vi "BoP Model Control.vi"() -> ()   [LabVIEW 2017]
uses:
  <vilib>/Platform/TimedLoop/XDataNode/timing_clust.ctl
  <vilib>/Platform/TimedLoop/XDataNode/nitl_modes.ctl
  <vilib>/Platform/TimedLoop/XDataNode/wakeup.ctl
  <vilib>/Model Interface Toolkit/Model Interface Toolkit.lvclass/Model Interface Toolkit.ctl
  <vilib>/Model Interface Toolkit/Model Update.vi
  <vilib>/Model Interface Toolkit/Tick Model.vi
  <vilib>/Model Interface Toolkit/Probe Signals.vi
  <vilib>/Model Interface Toolkit/Multirate/Dispatch Model Tasks.vi
  <vilib>/Model Interface Toolkit/Call Model Start Routine.vi
  <vilib>/Model Interface Toolkit/Handle Error.vi
  <vilib>/Model Interface Toolkit/Multirate/Wait on Tasks.vi
  <vilib>/Model Interface Toolkit/Check Error.vi
  <vilib>/Model Interface Toolkit/Generate Error Cluster.vi
  <vilib>/Platform/TimedLoop/scheduler/LVUserAPI/Fire Software-Triggered Timing Source.vi
  <vilib>/Platform/TimedLoop/XDataNode/XDataNode.xnode
  <vilib>/Model Interface Toolkit/Model Interface Toolkit.lvclass
  <vilib>/Platform/TimedLoop/XDataNode/XDNodeRunTimeDep.lvlib
panel:
  in  "Stop":bool=TRUE
  in  "Model Path":path
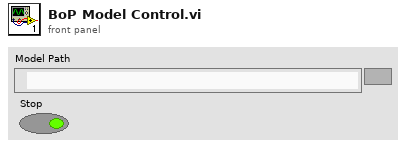
[diagram p1: front panel]
types:
  T1 = typedef "XDNodeRunTimeDep.lvlib/timing_clust.ctl" = cluster{"Expected End [f-1]":u64, "Actual End [f-1]":u64, "Finished Late? [f-1]":bool, "Expected End [i-1]":u64, "Actual End [i-1]":u64, "Finished Late? [i-1]":bool, "Expected Start [i]":u64, "Actual Start [i]":u64, "Expected Start [f]":u64, "Actual Start [f]":u64, "Source Name":string, "Structure Name":string, "Period":i64, "Deadline":i64, "Offset":i64, "Start":i64, "Priority":i32, "Timeout":i32, "Mode":T2, "Wakeup Reason":T3, "Error":errorcluster, "Source Type":string, "Secondary Source Type":string, "Global End Time":u64, "Global Start Time":u64, "Frame Duration":u64, "Iteration Duration":u64, "Assigned CPU":i32, "I/O Scan Engine Mode":u32}
  T2 = typedef "XDNodeRunTimeDep.lvlib/nitl_modes.ctl" = enum32{"No Change", "Process missed periods, maintain original phase", "Discard missed periods, maintain original phase", "Process missed periods, ignore original phase", "Discard missed periods, ignore original phase"}
  T3 = typedef "XDNodeRunTimeDep.lvlib/wakeup.ctl" = enum32{"Normal", "Aborted", "Asynchronous wakeup", "Timing source error", "Timed loop error", "Timeout"}
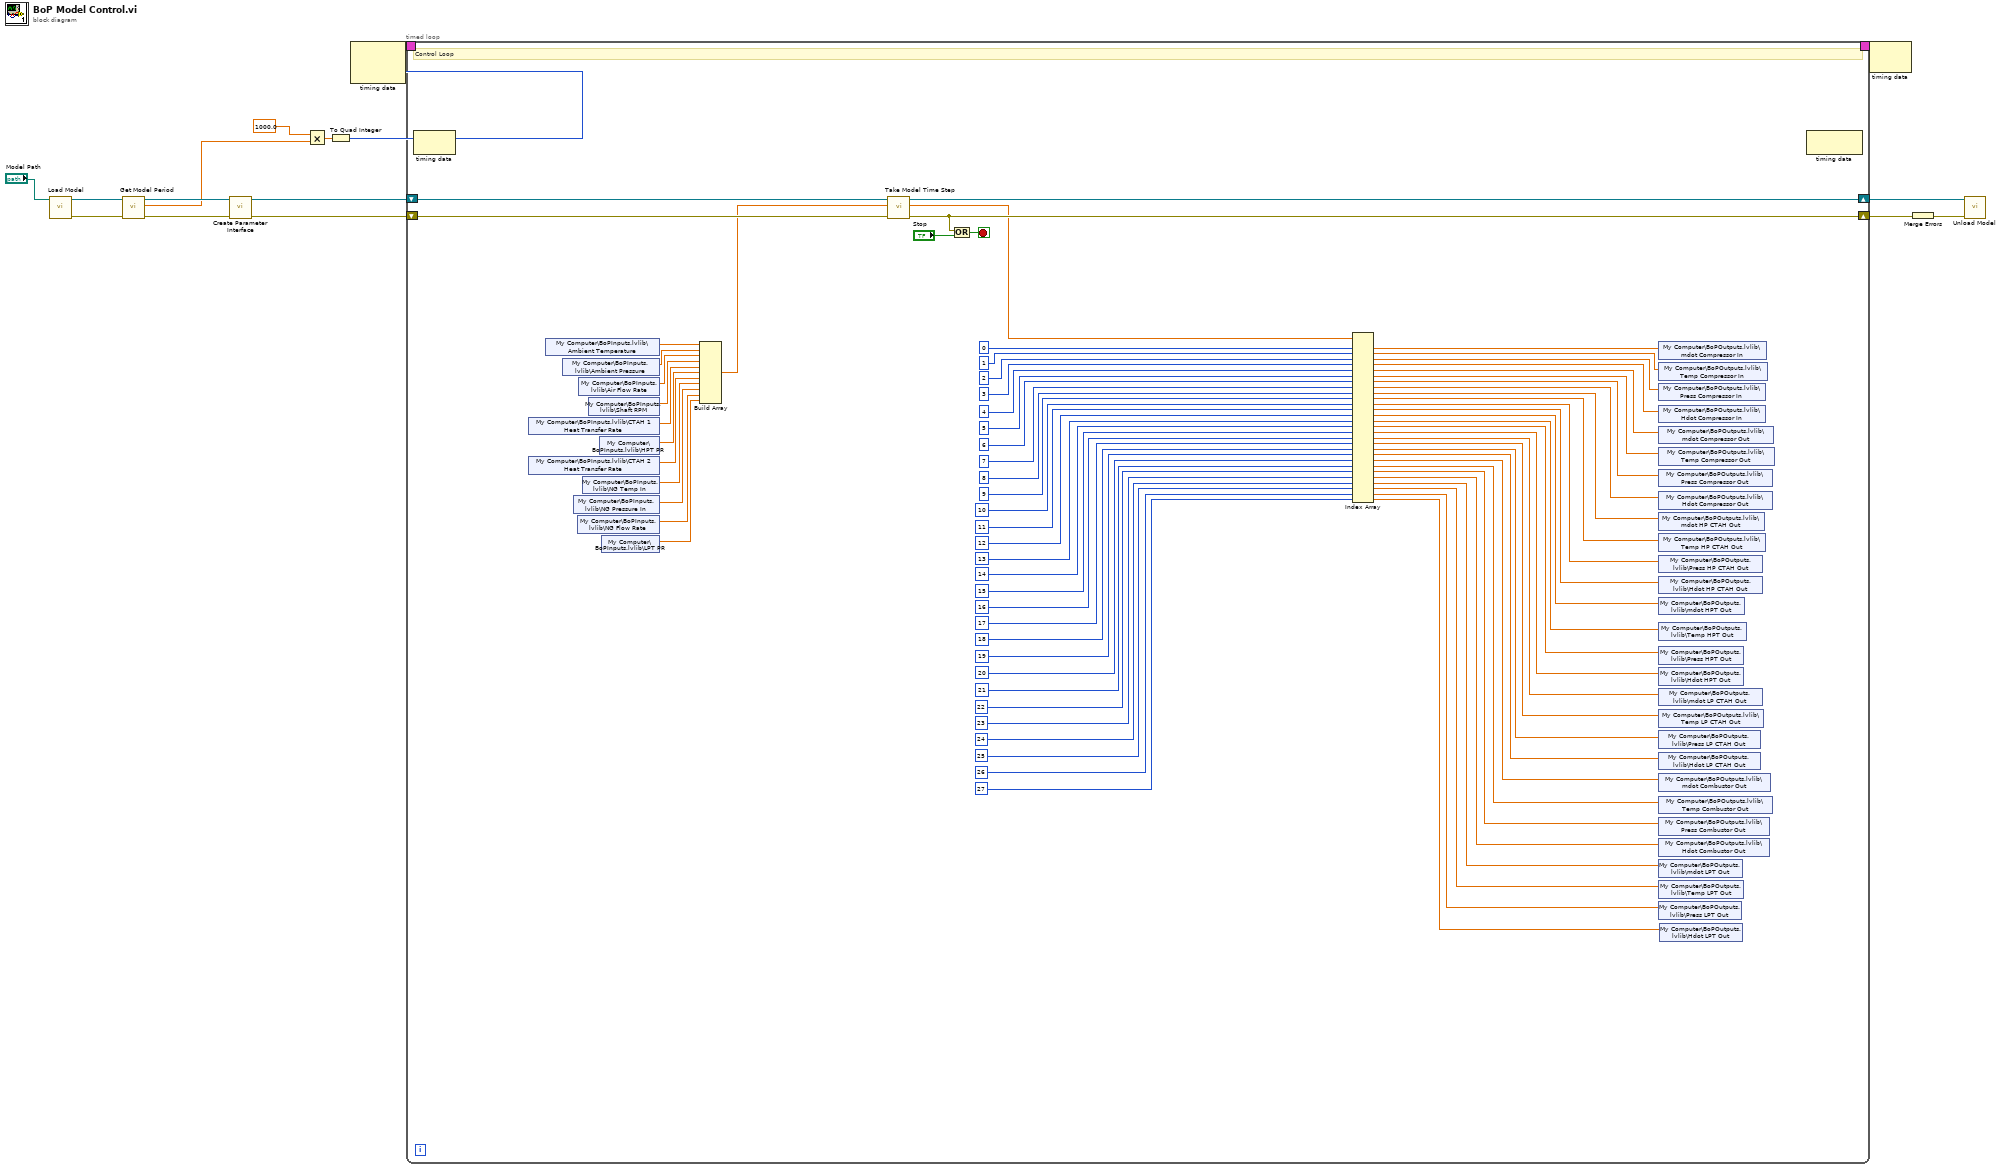
[diagram p0: block diagram]
diagram:
  n1 = call <vilib>:"Load Model.vi"("Model Path"="Model Path") -> ("error out"=w10:errorcluster, "Model out"=w13:refnum<class "Model Interface Toolkit.lvclass">)  [unwired: 9 in]
  n2 = call <vilib>:"Get Model Period.vi"("error in"=w10, "Model in"=w13) -> ("error out"=w9:errorcluster, "Model Period (s)"=w3:dbl, "Model out"=w12:refnum<class "Model Interface Toolkit.lvclass">)  [unwired: 7 in]
  n3 = call <vilib>:"Create Parameter Interface.vi"("error in"=w9, "Model in"=w12) -> ("error out"=w8:errorcluster, "Model out"=w11:refnum<class "Model Interface Toolkit.lvclass">)  [unwired: 7 in, 1 out]
  n4 = Multiply(x=1000.0, y=w3) -> (x*y=w2:dbl)
  n5 = To Quad Integer(1:w2) -> (0:w1:i64)
  n6 = node-c288(w1) -> (w15:T1)  [unwired: 1 in]
  n7 = timed-loop {
    timing: w15 -> [_]
    timing-out: [_] -> w14
    shift-right: [w90] -> w7
    shift-left: w11 -> [w91]
    shift-right: [w87] -> w6
    shift-left: w8 -> [w89]
    stop <- w88 stop-if-true
    # "Control Loop"
    n8 = node-c288() -> ()  [unwired: 1 in, 1 out]
    n9 = shared-variable "My Computer\\BoPInputs.lvlib\\CTAH 1 Heat Transfer Rate"() -> (w79:sgl)  [unwired: 1 in, 1 out]
    n10 = shared-variable "My Computer\\BoPInputs.lvlib\\CTAH 2 Heat Transfer Rate"() -> (w77:sgl)  [unwired: 1 in, 1 out]
    n11 = shared-variable "My Computer\\BoPInputs.lvlib\\Ambient Temperature"() -> (w83:sgl)  [unwired: 1 in, 1 out]
    n12 = shared-variable "My Computer\\BoPInputs.lvlib\\Ambient Pressure"() -> (w82:sgl)  [unwired: 1 in, 1 out]
    n13 = shared-variable "My Computer\\BoPInputs.lvlib\\NG Pressure In"() -> (w75:sgl)  [unwired: 1 in, 1 out]
    n14 = shared-variable "My Computer\\BoPInputs.lvlib\\NG Flow Rate"() -> (w74:sgl)  [unwired: 1 in, 1 out]
    n15 = shared-variable "My Computer\\BoPInputs.lvlib\\Air Flow Rate"() -> (w81:sgl)  [unwired: 1 in, 1 out]
    n16 = shared-variable "My Computer\\BoPInputs.lvlib\\NG Temp In"() -> (w76:sgl)  [unwired: 1 in, 1 out]
    n17 = shared-variable "My Computer\\BoPInputs.lvlib\\Shaft RPM"() -> (w80:sgl)  [unwired: 1 in, 1 out]
    n18 = shared-variable "My Computer\\BoPInputs.lvlib\\HPT PR"() -> (w78:sgl)  [unwired: 1 in, 1 out]
    n19 = shared-variable "My Computer\\BoPInputs.lvlib\\LPT PR"() -> (w73:sgl)  [unwired: 1 in, 1 out]
    n20 = Build Array(w83, w82, w81, w80, w79, w78, w77, w76, w75, w74, w73) -> (w86:sgl[])
    n21 = call <vilib>:"Take Model Time Step.vi"("error in (no error)"=w89, "Inport Array"=w86, "Model in"=w91) -> ("error out"=w87:errorcluster, "Outport Array out"=w85:dbl[], "Model out"=w90:refnum<class "Model Interface Toolkit.lvclass">)  [unwired: 6 in]
    n22 = Or(x=w87, y="Stop") -> (x .or. y?=w88:bool)
    n23 = Index Array(array=w85, index #1=0 ("index"), index #2=1 ("index"), index #3=2 ("index"), index #4=3 ("index"), index #5=4 ("index"), index #6=5 ("index"), index #7=6 ("index"), index #8=7 ("index"), index #9=8 ("index"), index #10=9 ("index"), index #11=10 ("index"), index #12=11 ("index"), index #13=12 ("index"), index #14=13 ("index"), index #15=14 ("index"), index #16=15 ("index"), index #17=16 ("index"), index #18=17 ("index"), index #19=18 ("index"), index #20=19 ("index"), index #21=20 ("index"), index #22=21 ("index"), index #23=22 ("index"), index #24=23 ("index"), index #25=24 ("index"), index #26=25 ("index"), index #27=26 ("index"), index #28=27 ("index")) -> (element #1=w44:dbl, element #2=w43:dbl, element #3=w42:dbl, element #4=w41:dbl, element #5=w40:dbl, element #6=w39:dbl, element #7=w38:dbl, element #8=w37:dbl, element #9=w36:dbl, element #10=w35:dbl, element #11=w34:dbl, element #12=w33:dbl, element #13=w32:dbl, element #14=w31:dbl, element #15=w30:dbl, element #16=w29:dbl, element #17=w28:dbl, element #18=w27:dbl, element #19=w26:dbl, element #20=w25:dbl, element #21=w24:dbl, element #22=w23:dbl, element #23=w22:dbl, element #24=w21:dbl, element #25=w20:dbl, element #26=w19:dbl, element #27=w18:dbl, element #28=w17:dbl)
    n24 = shared-variable "My Computer\\BoPOutputs.lvlib\\mdot Compressor In"(w44) -> ()  [unwired: 1 in, 1 out]
    n25 = shared-variable "My Computer\\BoPOutputs.lvlib\\Temp Compressor In"(w43) -> ()  [unwired: 1 in, 1 out]
    n26 = shared-variable "My Computer\\BoPOutputs.lvlib\\Press Compressor In"(w42) -> ()  [unwired: 1 in, 1 out]
    n27 = shared-variable "My Computer\\BoPOutputs.lvlib\\Hdot Compressor In"(w41) -> ()  [unwired: 1 in, 1 out]
    n28 = shared-variable "My Computer\\BoPOutputs.lvlib\\mdot Compressor Out"(w40) -> ()  [unwired: 1 in, 1 out]
    n29 = shared-variable "My Computer\\BoPOutputs.lvlib\\Temp Compressor Out"(w39) -> ()  [unwired: 1 in, 1 out]
    n30 = shared-variable "My Computer\\BoPOutputs.lvlib\\Press Compressor Out"(w38) -> ()  [unwired: 1 in, 1 out]
    n31 = shared-variable "My Computer\\BoPOutputs.lvlib\\Hdot Compressor Out"(w37) -> ()  [unwired: 1 in, 1 out]
    n32 = shared-variable "My Computer\\BoPOutputs.lvlib\\mdot HP CTAH Out"(w36) -> ()  [unwired: 1 in, 1 out]
    n33 = shared-variable "My Computer\\BoPOutputs.lvlib\\Temp HP CTAH Out"(w35) -> ()  [unwired: 1 in, 1 out]
    n34 = shared-variable "My Computer\\BoPOutputs.lvlib\\Press HP CTAH Out"(w34) -> ()  [unwired: 1 in, 1 out]
    n35 = shared-variable "My Computer\\BoPOutputs.lvlib\\Hdot HP CTAH Out"(w33) -> ()  [unwired: 1 in, 1 out]
    n36 = shared-variable "My Computer\\BoPOutputs.lvlib\\mdot HPT Out"(w32) -> ()  [unwired: 1 in, 1 out]
    n37 = shared-variable "My Computer\\BoPOutputs.lvlib\\Temp HPT Out"(w31) -> ()  [unwired: 1 in, 1 out]
    n38 = shared-variable "My Computer\\BoPOutputs.lvlib\\Press HPT Out"(w30) -> ()  [unwired: 1 in, 1 out]
    n39 = shared-variable "My Computer\\BoPOutputs.lvlib\\Hdot HPT Out"(w29) -> ()  [unwired: 1 in, 1 out]
    n40 = shared-variable "My Computer\\BoPOutputs.lvlib\\mdot LP CTAH Out"(w28) -> ()  [unwired: 1 in, 1 out]
    n41 = shared-variable "My Computer\\BoPOutputs.lvlib\\Temp LP CTAH Out"(w27) -> ()  [unwired: 1 in, 1 out]
    n42 = shared-variable "My Computer\\BoPOutputs.lvlib\\Press LP CTAH Out"(w26) -> ()  [unwired: 1 in, 1 out]
    n43 = shared-variable "My Computer\\BoPOutputs.lvlib\\Hdot LP CTAH Out"(w25) -> ()  [unwired: 1 in, 1 out]
    n44 = shared-variable "My Computer\\BoPOutputs.lvlib\\mdot Combustor Out"(w24) -> ()  [unwired: 1 in, 1 out]
    n45 = shared-variable "My Computer\\BoPOutputs.lvlib\\Temp Combustor Out"(w23) -> ()  [unwired: 1 in, 1 out]
    n46 = shared-variable "My Computer\\BoPOutputs.lvlib\\Press Combustor Out"(w22) -> ()  [unwired: 1 in, 1 out]
    n47 = shared-variable "My Computer\\BoPOutputs.lvlib\\Hdot Combustor Out"(w21) -> ()  [unwired: 1 in, 1 out]
    n48 = shared-variable "My Computer\\BoPOutputs.lvlib\\mdot LPT Out"(w20) -> ()  [unwired: 1 in, 1 out]
    n49 = shared-variable "My Computer\\BoPOutputs.lvlib\\Temp LPT Out"(w19) -> ()  [unwired: 1 in, 1 out]
    n50 = shared-variable "My Computer\\BoPOutputs.lvlib\\Press LPT Out"(w18) -> ()  [unwired: 1 in, 1 out]
    n51 = shared-variable "My Computer\\BoPOutputs.lvlib\\Hdot LPT Out"(w17) -> ()  [unwired: 1 in, 1 out]
    n52 = node-c288() -> ()  [unwired: 1 in, 1 out]
  }
  n53 = node-c288(w14) -> ()  [unwired: 1 out]
  n54 = Merge Errors(w6) -> (w5:errorcluster)
  n55 = call <vilib>:"Unload Model.vi"("error in (no error)"=w5, "Model in"=w7) -> ()  [unwired: 9 in, 1 out]
